vi "DMR_CloseDevice.vi"(4 "device handle IN":i32, 5 "driver handle IN":i32) -> (0 "error code OUT":i32, 1 "device handle OUT":i32)   [LabVIEW 2010]
doc: "Closes a device.\n\nThis VI will try to close a device previously initialised by a call to \nDMR_OpenDevice. The device handle (obtained from the DMR_GetDevice VI) and the driver handle(obtained from the DMR_OpenDevice VI) must be passed to the input terminals.\n\nOnce this VI has been executed, every device driver object handle (e.g. list handles or handles to certain properties) for this device will become invalid.\n\nSee also:\nDMR_OpenDevice,\nDMR_GetDevice\n\nThe error code OUT terminal will deliver 0 if successful or a negative error code otherwise. A list of valid error codes and their meaning can be found in the manual about this interface."
uses:
  mvDeviceManager.dll
panel:
  # "OUTPUT"
  # "INPUT"
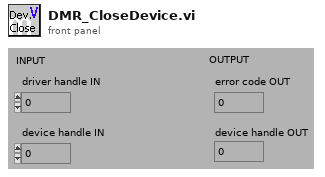
[diagram p1: front panel]
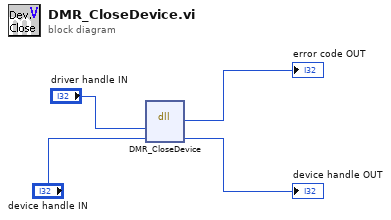
[diagram p0: block diagram]
diagram:
  n1 = dll-call lib="mvDeviceManager.dll" fn="DMR_CloseDevice"("hDrv"="driver handle IN", "hDev"="device handle IN") -> (→"error code OUT":i32, "hDev"=→"device handle OUT":i32)  [unwired: 4 in, 2 out]
